vi "etc_XCITE_ExecuteCommandWithValue.vi"(8 "error in (no error)":errorcluster {"code" format="%x"}, 9 "in_value":string, 10 "command":string, 11 "h":u64) -> (0 "error out":errorcluster {"code" format="%x"}, 1 "answer":string, 2 "ErrorMessage":i32 format="%x", 3 "h out":u64)   [LabVIEW 2019, in "XCite.lvlib"]
doc: "Sends a command to execute on the slelected X-cite device."
uses:
  XCite.lvlib
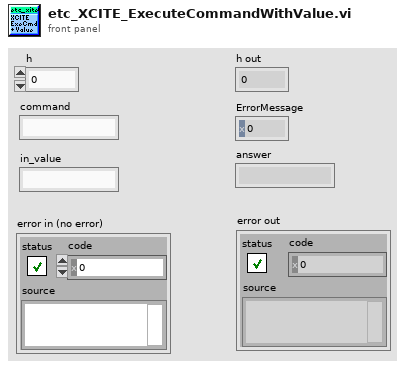
[diagram p1: front panel]
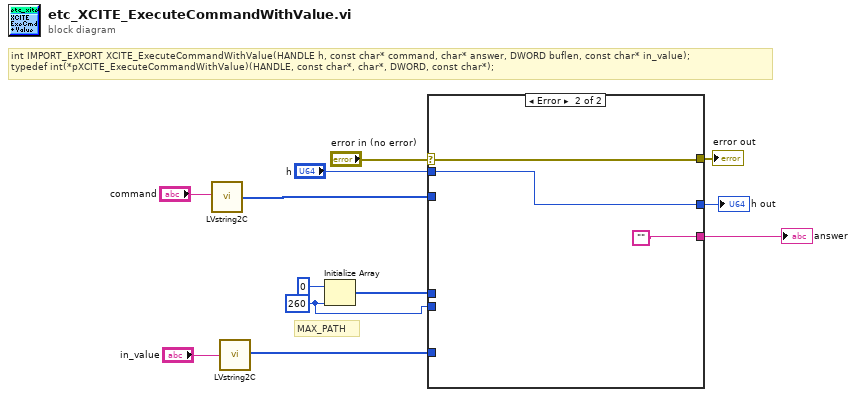
[diagram p0: block diagram]
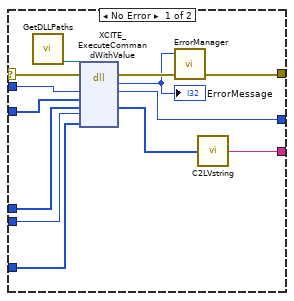
[diagram p2: hidden frame]
diagram:
  w5 = u16 260 ("dimension size")
  # "MAX_PATH"
  # "int IMPORT_EXPORT XCITE_ExecuteCommandWithValue(HANDLE h, const char* command, char* answer, DWORD buflen, const char* in_value);\ntypedef int(*pXCITE_ExecuteCommandWithValue)(HANDLE, const char*, char*, DWORD, const char*);"
  n1 = call "LVstring2C.vi"("LVString"="command") -> ("CString"=w4:u8[])  [unwired: 3 in, 1 out]
  n2 = call "LVstring2C.vi"("LVString"="in_value") -> ("CString"=w2:u8[])  [unwired: 3 in, 1 out]
  n3 = Initialize Array(u8 0, w5) -> (w6:u8[])
  n4 = case shown="Error" "error in (no error)" {
    selector: "error in (no error)" -> [w25 w28]
    tunnel: [w23 w28] -> w12
    tunnel: "h" -> [w21 w27]
    tunnel: [w20 w27] -> w10
    tunnel: w5 -> [w18 _]
    tunnel: [w13 ""] -> w8
    tunnel: w6 -> [w17 _]
    tunnel: w2 -> [w16 _]
    tunnel: w4 -> [w15 _]
    frame No Error {
      n5 = call "GetDLLPaths.vi"() -> ("etc_xcite_path"=w19:path)  [unwired: 8 in, 3 out]
      n6 = dll-call lib="C:/LabVIEWDevFall2024/pco.labview/labview_sdk/runtime/bin64/etc_xcite.dll" fn="XCITE_ExecuteCommandWithValue"(path in=w19, error in=w25, "h"=w21, "command"=w15, "answer"=w17, "buflen"=w18, "in_value"=w16) -> (error out=w24:errorcluster, "return type"=w22:i32, "h"=w20:u64, "answer"=w14:u8[])  [unwired: 4 in, 1 out]
      "ErrorMessage" <- w22
      n7 = call "ErrorManager.vi"("error in (no error)"=w24, "error code"=w22) -> ("error out"=w23:errorcluster)  [unwired: 2 in, 1 out]
      n8 = call "C2LVstring.vi"("CString"=w14) -> ("LVString"=w13:string)  [unwired: 4 in]
    }
    frame Error {
    }
  }
  "error out" <- w12
  "h out" <- w10
  "answer" <- w8
